vi "OCR_Main_Function.vi"(8 "error in (no error)":errorcluster, 9 "Item Names":string[](array[string]), 10 "String":string, 11 "Refnum in":T1) -> (0 "error out":errorcluster)   [LabVIEW 2019]
uses:
  <vilib>/vision/Image Controls.llb/IMAQ Image.ctl
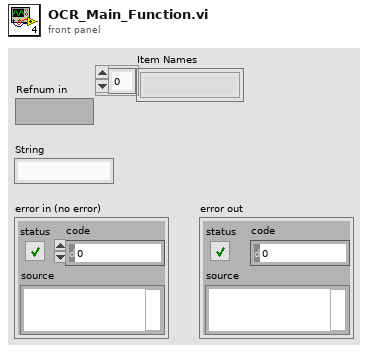
[diagram p1: front panel]
types:
  T1 = typedef "IMAQ Image.ctl" = refnum<image>
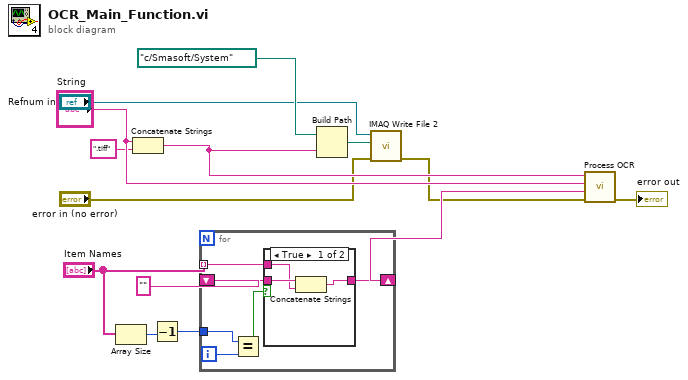
[diagram p0: block diagram]
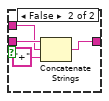
[diagram p2: hidden frame]
diagram:
  n1 = Array Size(array="Item Names") -> (size(s)=w2:i32)
  n2 = Concatenate Strings("String", ".tiff" ("string")) -> (w10:string)
  n3 = Decrement(x=w2) -> (x-1=w1:i32)
  n4 = for {
    tunnel: "Item Names" -> [w19] mode=indexing
    shift-right: [w18] -> w13
    shift-left: "" -> [w20]
    tunnel: w1 -> [w16]
    i -> [w17]
    n5 = Equal?(x=w16, y=w17) -> (x = y?=w15:bool)
    n6 = case shown="True" w15 {
      tunnel: w20 -> [w23 w27]
      tunnel: w19 -> [w22 w26]
      tunnel: [w21 w25] -> w18
      frame True {
        n7 = Concatenate Strings(w23, w22) -> (w21:string)
      }
      frame False {
        n8 = Concatenate Strings(w27, w26, "+" ("string")) -> (w25:string)
      }
    }
  }
  n9 = Build Path(base path=path "c:/Smasoft/System", name or relative path=w10) -> (appended path=w11:path)
  n10 = call-poly "IMAQ Write File 2"("error in (no error)"="error in (no error)", "File Path"=w11, "Image"="Refnum in") -> ("error out"=w4:errorcluster)  [unwired: 7 in, 1 out]
  n11 = call "Process OCR.vi"("error in (no error)"=w4, "Language"=w13, "Output File Name"="String", "Image Name"=w10) -> ("error out"=→"error out":errorcluster)  [unwired: 7 in]
